vi "Grabber.vi"   [LabVIEW 2014]
uses:
  Begin/Global RefNums.vi
  Begin/Global Variables.vi
  <vilib>/Rock Robotics/WPI/Solenoid/Deprecated/WPI_SolenoidSetBool.vi
types:
  T1 = typedef "WPI_SolenoidDevRef.ctl" = cluster{"DevStatus":errorcluster, "Pneumatics Control Module":u8, "Forward Solenoid Channel":T2, "Reverse Solenoid Channel":T2}
  T2 = typedef "WPI_SolenoidChannel.ctl" = enum8{"Solenoid 0", "Solenoid 1", "Solenoid 2", "Solenoid 3", "Solenoid 4", "Solenoid 5", "Solenoid 6", "Solenoid 7", "Invalid"}
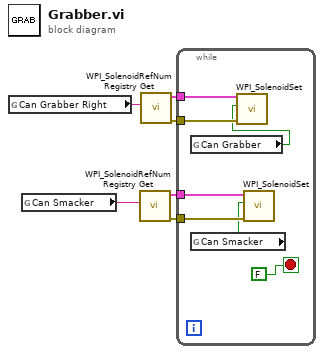
[diagram p0: block diagram]
diagram:
  n1 = global read "Global RefNums.vi" "Can Grabber Right"() -> (w6:string)
  n2 = global read "Global RefNums.vi" "Can Smacker"() -> (w1:string)
  n3 = call <vilib>:"WPI_SolenoidRefNum Registry Get.vi"("refnum name"=w1) -> ("error out"=w3:errorcluster, "SolenoidDevRef"=w2:T1)  [unwired: 9 in]
  n4 = call <vilib>:"WPI_SolenoidRefNum Registry Get.vi"("refnum name"=w6) -> ("error out"=w4:errorcluster, "SolenoidDevRef"=w5:T1)  [unwired: 9 in]
  n5 = while {
    tunnel: w5 -> [w12]
    tunnel: w4 -> [w11]
    tunnel: w2 -> [w8]
    tunnel: w3 -> [w9]
    stop <- FALSE stop-if-true
    n6 = global read "Global Variables.vi" "Can Grabber"() -> (w10:bool)
    n7 = global read "Global Variables.vi" "Can Smacker"() -> (w7:bool)
    n8 = call-poly <vilib>:"WPI_SolenoidSet.vi"("error in (no error)"=w11, "Value"=w10, "SolenoidDevRef"=w12) -> ()  [unwired: 7 in, 2 out]
    n9 = call-poly <vilib>:"WPI_SolenoidSet.vi"("error in (no error)"=w9, "Value"=w7, "SolenoidDevRef"=w8) -> ()  [unwired: 7 in, 2 out]
  }
